vi "Start.vi"(8 "error in (no error)":errorcluster, 10 "Variant":variant, 11 "FFT in":refnum<class "FFT.lvclass">) -> (0 "error out":errorcluster, 3 "FFT out":refnum<class "FFT.lvclass">)   [LabVIEW 2018, in "AnalysisPlugins.lvlib" / "FFT.lvclass"]
uses:
  FFT.lvclass
  C:/projects/ICDAS/NistPluggableModules/Analysis/AnalysisPlugins/AnalysisPluginBaseClass/AnalysisPluginsBase.lvclass
  AnalysisPluginBaseClass/Typedefs/SampleDataInput.ctl
  AnalysisPluginBaseClass/AnalysisPluginsBase.lvclass/AnalysisPluginsBase.ctl
  AnalysisPluginBaseClass/Accessors/Read SampleDataQueName.vi
  AnalysisPluginBaseClass/Accessors/Write AnalysisTime.vi
  FitterBaseClass/FitterBase.lvclass
  AnalysisPluginBaseClass/AnalysisPluginsBase.lvclass
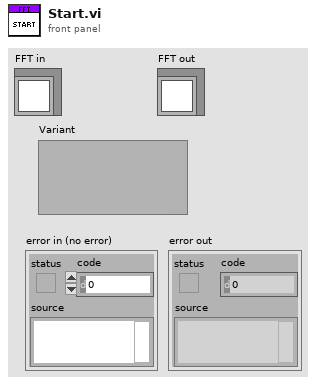
[diagram p1: front panel]
types:
  T1 = typedef "AnalysisPlugins.lvlib/AnalysisPluginsBase.lvclass/SampleDataInput.ctl" = waveform(dbl)[]
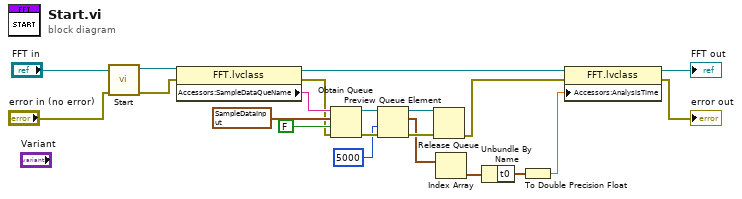
[diagram p0: block diagram]
diagram:
  n1 = call-parent "Start.vi"("error in (no error)"="error in (no error)", "FitterBase in"="FFT in") -> ("error out"=w3:errorcluster, "FitterBase out"=w5:refnum<class "FFT.lvclass">)  [unwired: 8 in]
  n2 = property class="FFT.lvclass"(reference=w5, error in=w3) -> (reference out=w19:refnum<class "FFT.lvclass">, error out=w15:errorcluster, "Accessors:SampleDataQueName"=w16:string)
  n3 = Obtain Queue(name (unnamed)=w16, element data type=T1 [{"t0"=timestamp(0 s since 1904-01-01), "dt"=1.0, "Y"=[]}] ("clSampleDataArray"), create if not found? (T)=FALSE, error in (no error)=w15) -> (queue out=w13:refnum<queue>, error out=w14:errorcluster)  [unwired: 1 in, 1 out]
  n4 = Preview Queue Element(queue=w13, timeout in ms (-1)=5000, error in (no error)=w14) -> (queue out=w12:refnum<queue>, element=w10:T1, error out=w11:errorcluster)  [unwired: 1 out]
  n5 = Release Queue(queue=w12, error in (no error)=w11) -> (error out=w1:errorcluster)  [unwired: 1 in, 2 out]
  n6 = Index Array(array=w10) -> (element=w9:waveform(dbl))  [unwired: 1 in]
  n7 = Unbundle By Name(w9) -> ("t0"=w8:timestamp)
  n8 = To Double Precision Float(number=w8) -> (double precision float=w7:dbl)
  n9 = property class="FFT.lvclass"(reference=w19, error in=w1, "Accessors:AnalysisTime"=w7) -> (reference out=→"FFT out":refnum<class "FFT.lvclass">, error out=→"error out":errorcluster)
